vi "Create Coverage Report - Line Rate is Covered over Total.vi"() -> ()   [LabVIEW 2017, in "Cobertura.Tests.lvlib"]
uses:
  Cobertura.Tests.lvlib
  Cobertura/Coverage/Coverage.lvclass/Coverage.ctl
  Cobertura/Package/Package.lvclass/Package.ctl
  Cobertura/Class/Class.lvclass/Class.ctl
  Cobertura/Method/Method.lvclass/Method.ctl
  Cobertura/Coverage/Read Packages.vi
  Cobertura/Package/Read Classes.vi
  Cobertura/Class/Read Methods.vi
  Cobertura/Method/Read Line Rate.vi
  Fake Project Inspector/Fake Project Inspector.lvclass
  C:/Users/Pascal/Projects/Home/lvunit/Cobertura/Project Inspector Base/Project Inspector Base.lvclass
  Fake Code Coverage/Fake Code Coverage.lvclass
  C:/Users/Pascal/Projects/Home/lvunit/Code Coverage/Code Coverage.lvclass
  Fake Code Inspector/Fake Code Inspector.lvclass
  C:/Users/Pascal/Projects/Home/lvunit/Cobertura/Code Inspector Base/Code Inspector Base.lvclass
  Cobertura/Package/Package.lvclass
  Cobertura/Class/Class.lvclass
  Cobertura/Method/Method.lvclass
  Cobertura/Cobertura.lvlib
  <vilib>/PNR/Transparent Assertions/Transparent Assertions/Transparent Assertions.lvlib
  Cobertura/Coverage/Coverage.lvclass
panel:
  out "error out":errorcluster
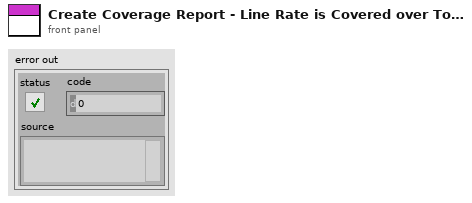
[diagram p1: front panel]
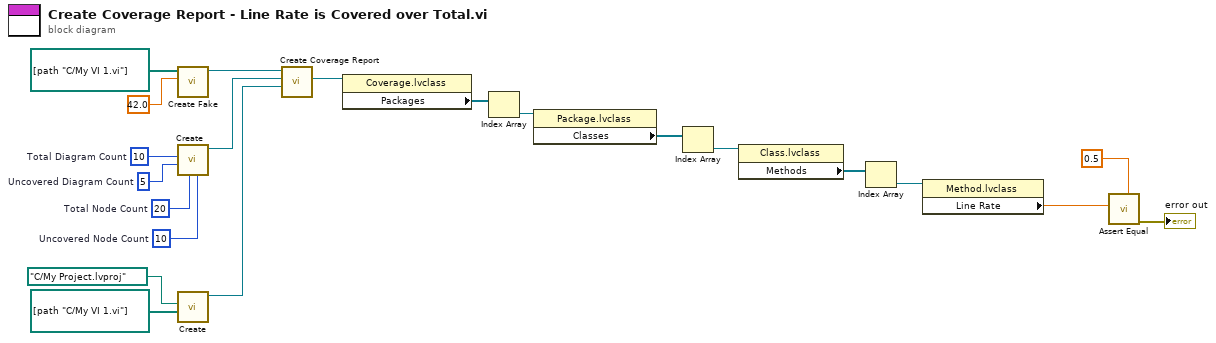
[diagram p0: block diagram]
diagram:
  w1 = 10  # Uncovered Node Count
  w2 = 20  # Total Node Count
  w3 = 5  # Uncovered Diagram Count
  w4 = 10  # Total Diagram Count
  n1 = call "Create Fake.vi"("Coverage Percentage"=42.0, "All VIs Measured"=path[] [path "C:/My VI 1.vi"] ("Item Paths")) -> ("Fake Code Coverage"=w9:refnum<class "Fake Code Coverage.lvclass">)  [unwired: 8 in, 1 out]
  n2 = call "Create.vi"("Uncovered Node Count"=w1, "Total Node Count"=w2, "Uncovered Diagram Count"=w3, "Total Diagram Count"=w4) -> ("Fake Code Inspector"=w5:refnum<class "Fake Code Inspector.lvclass">)  [unwired: 6 in, 1 out]
  n3 = call "Create.vi"("Item Paths"=path[] [path "C:/My VI 1.vi"], "Path"=path "C:/My Project.lvproj") -> ("Fake Project Inspector"=w18:refnum<class "Fake Project Inspector.lvclass">)  [unwired: 8 in, 1 out]
  n4 = call "Create Coverage Report.vi"("Project Inspector"=w18, "Code Inspector"=w5, "CodeCoverage in"=w9) -> ("Coverage"=w21:refnum<class "Coverage.lvclass">)  [unwired: 7 in, 1 out]
  n5 = property class="Coverage.lvclass"(reference=w21) -> ("Packages"=w19:refnum<class "Package.lvclass">[])  [unwired: 1 in, 2 out]
  n6 = Index Array(array=w19) -> (element=w16:refnum<class "Package.lvclass">)  [unwired: 1 in]
  n7 = property class="Package.lvclass"(reference=w16) -> ("Classes"=w15:refnum<class "Class.lvclass">[])  [unwired: 1 in, 2 out]
  n8 = Index Array(array=w15) -> (element=w13:refnum<class "Class.lvclass">)  [unwired: 1 in]
  n9 = property class="Class.lvclass"(reference=w13) -> ("Methods"=w12:refnum<class "Method.lvclass">[])  [unwired: 1 in, 2 out]
  n10 = Index Array(array=w12) -> (element=w11:refnum<class "Method.lvclass">)  [unwired: 1 in]
  n11 = property class="Method.lvclass"(reference=w11) -> ("Line Rate"=w10:dbl)  [unwired: 1 in, 2 out]
  n12 = call <vilib>:"Assert Equal.vi"("Expected"=0.5 ("Branch Rate"), "Actual"=w10) -> ("error out"=→"error out":errorcluster)  [unwired: 9 in]
